vi "Create RxTx.vi"(8 "error in (no error)":errorcluster, 10 "Remote IP":string="200.131.64.49", 11 "Channel GUI in":refnum<class "Channel.lvclass">) -> (0 "error out":errorcluster, 3 "Channel GUI out":refnum<class "Channel.lvclass">)   [LabVIEW 2018, in "Channel.lvclass"]
uses:
  Channel.lvclass
  Channel.lvclass/Channel.ctl
  RxTx/RxTx.lvclass
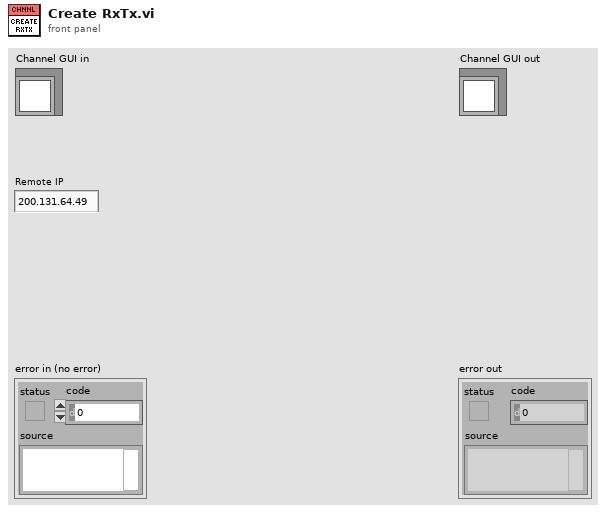
[diagram p1: front panel]
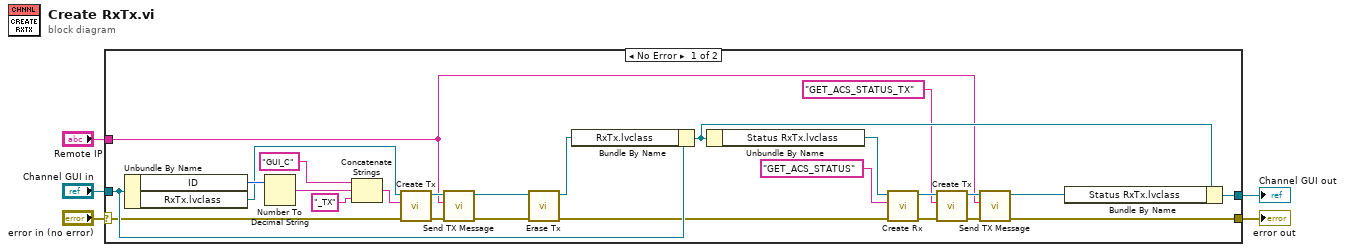
[diagram p0: block diagram]
diagram:
  n1 = case shown="No Error" "error in (no error)" {
    selector: "error in (no error)" -> [w26 w33]
    tunnel: [w10 w33] -> w3
    tunnel: [w21 w32] -> w2
    tunnel: "Channel GUI in" -> [w31 w32]
    tunnel: "Remote IP" -> [w8 _]
    frame No Error {
      n2 = Unbundle By Name(w31) -> ("ID"=w28:u8, "RxTx.lvclass"=w25:refnum<class "RxTx.lvclass">)
      n3 = Number To Decimal String(number=w28) -> (decimal integer string=w29:string)  [unwired: 1 in]
      n4 = Concatenate Strings("GUI_C", w29, "_TX") -> (w24:string)
      n5 = call "Create Tx.vi"("error in (no error)"=w26, "Writer Name"=w24, "RxTx in"=w25) -> ("error out"=w22:errorcluster, "RxTx out"=w23:refnum<class "RxTx.lvclass">)  [unwired: 7 in]
      n6 = call "Send TX Message.vi"("error in (no error)"=w22, "element"=w8, "RxTx in"=w23) -> ("error out"=w6:errorcluster, "RxTx out"=w7:refnum<class "RxTx.lvclass">)  [unwired: 7 in]
      n7 = call "Erase Tx.vi"("error in (no error)"=w6, "RxTx in"=w7) -> ("error out"=w12:errorcluster, "RxTx out"=w11:refnum<class "RxTx.lvclass">)  [unwired: 8 in]
      n8 = Bundle By Name(cluster=w31, "RxTx.lvclass"=w11) -> (w20:refnum<class "Channel.lvclass">)
      n9 = Unbundle By Name(w20) -> ("Status RxTx.lvclass"=w19:refnum<class "RxTx.lvclass">)
      n10 = call "Create Rx.vi"("error in (no error)"=w12, "Reader Name"="GET_ACS_STATUS" ("element"), "RxTx in"=w19) -> ("error out"=w17:errorcluster, "RxTx out"=w16:refnum<class "RxTx.lvclass">)  [unwired: 7 in]
      n11 = call "Create Tx.vi"("error in (no error)"=w17, "Writer Name"="GET_ACS_STATUS_TX" ("element"), "RxTx in"=w16) -> ("error out"=w13:errorcluster, "RxTx out"=w14:refnum<class "RxTx.lvclass">)  [unwired: 7 in]
      n12 = call "Send TX Message.vi"("error in (no error)"=w13, "element"=w8, "RxTx in"=w14) -> ("error out"=w10:errorcluster, "RxTx out"=w9:refnum<class "RxTx.lvclass">)  [unwired: 7 in]
      n13 = Bundle By Name(cluster=w20, "Status RxTx.lvclass"=w9) -> (w21:refnum<class "Channel.lvclass">)
    }
    frame Error {
    }
  }
  "error out" <- w3
  "Channel GUI out" <- w2
